vi "Round to Hundreths.vi"(4 "Raw":dbl) -> (1 "Rounded":dbl)   [LabVIEW 2021]
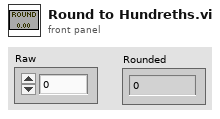
[diagram p1: front panel]
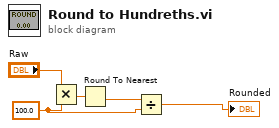
[diagram p0: block diagram]
diagram:
  w2 = 100.0 ("y")
  n1 = Multiply(x="Raw", y=w2) -> (x*y=w4:dbl)
  n2 = Round To Nearest(number=w4) -> (nearest integer value=w3:dbl)
  n3 = Divide(x=w3, y=w2) -> (x/y=→"Rounded":dbl)
